vi "ProbeMessageQueueDefault.vi"(11 "MessageQueue":refnum<class "MessageQueue.lvclass">) -> (2 "Value String":string, 3 "Boolean":bool)   [LabVIEW 2017, in "LapDog.Messaging.v3.lvlib" / "MessageQueue.lvclass"]
uses:
  MessageQueue.lvclass
  MessageQueue.lvclass/MessageQueue.ctl
  Message/Message.lvclass
panel:
  out "# Elements in Queue":i32
  out "Msgs":string[](array[string])
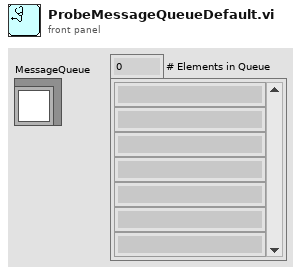
[diagram p1: front panel]
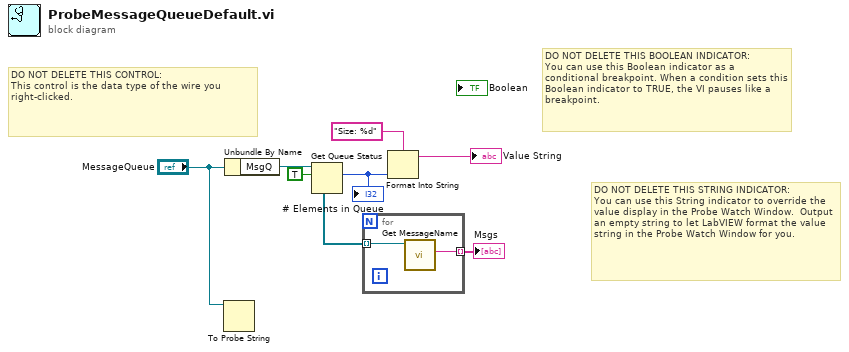
[diagram p0: block diagram]
diagram:
  # "DO NOT DELETE THIS STRING INDICATOR: \nYou can use this String indicator to override the value display in the Probe Watch Window.  Output an empty string to let LabVIEW format the value string in the Probe Watch Window for you."
  # "DO NOT DELETE THIS BOOLEAN INDICATOR: \nYou can use this Boolean indicator as a conditional breakpoint. When a condition sets this Boolean indicator to TRUE, the VI pauses like a breakpoint."
  # "DO NOT DELETE THIS CONTROL: \nThis control is the data type of the wire you right-clicked."
  n1 = To Probe String(7:"MessageQueue") -> ()  [unwired: 2 in, 2 out]
  n2 = Unbundle By Name("MessageQueue") -> ("MsgQ"=w7:refnum<queue>)
  n3 = Get Queue Status(queue=w7, return elements? (F)=TRUE) -> (# pending remove=w3:i32, elements=w5:refnum<class "Message.lvclass">[])  [unwired: 1 in, 6 out]
  "# Elements in Queue" <- w3
  n4 = for {
    tunnel: w5 -> [w10] mode=indexing
    tunnel: [w9] -> w4 mode=indexing
    n5 = call "Get MessageName.vi"("Message in"=w10) -> ("Message Name"=w9:string)  [unwired: 8 in, 2 out]
  }
  "Msgs" <- w4
  n6 = Format Into String(format string="Size: %d", w3) -> (resulting string=→"Value String":string)  [unwired: 2 in, 1 out]
